vi "SwerveMath_.vi"(2 "Rotation Multipliers":dbl, 3 "Trigger Axes/Turn Speed":cluster{"Left":dbl, "Right":dbl}, 4 "Strafe Multiplier":dbl, 5 "Angle (radians; 0 = right)":dbl, 6 "FieldCentric? (T)":bool=TRUE, 7 "Strafe Joystick Axes":cluster{"X":dbl, "Y":dbl}) -> (0 "Motor Angles":dbl[](array[numeric]), 1 "Motor Speeds":dbl[](array[numeric]))   [LabVIEW 2015]
uses:
  Swerve Drive Published Globals.vi
panel:
  in  "Rotation Angle Cluster":dbl
  in  "Rotation Multiplier":dbl
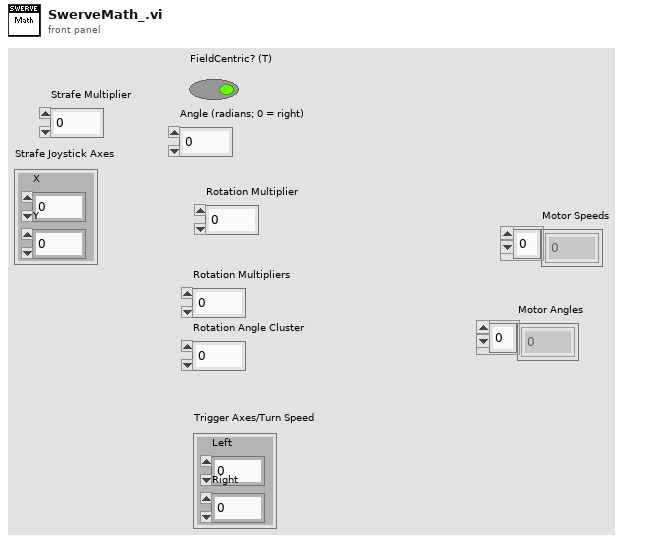
[diagram p1: front panel]
types:
  T1 = cluster{"FL Angle":dbl, "FR Angle":dbl, "RL Angle":dbl, "RR Angle":dbl}
  T2 = cluster{"normalized array[0]":dbl, "normalized array[1]":dbl, "normalized array[2]":dbl, "normalized array[3]":dbl}
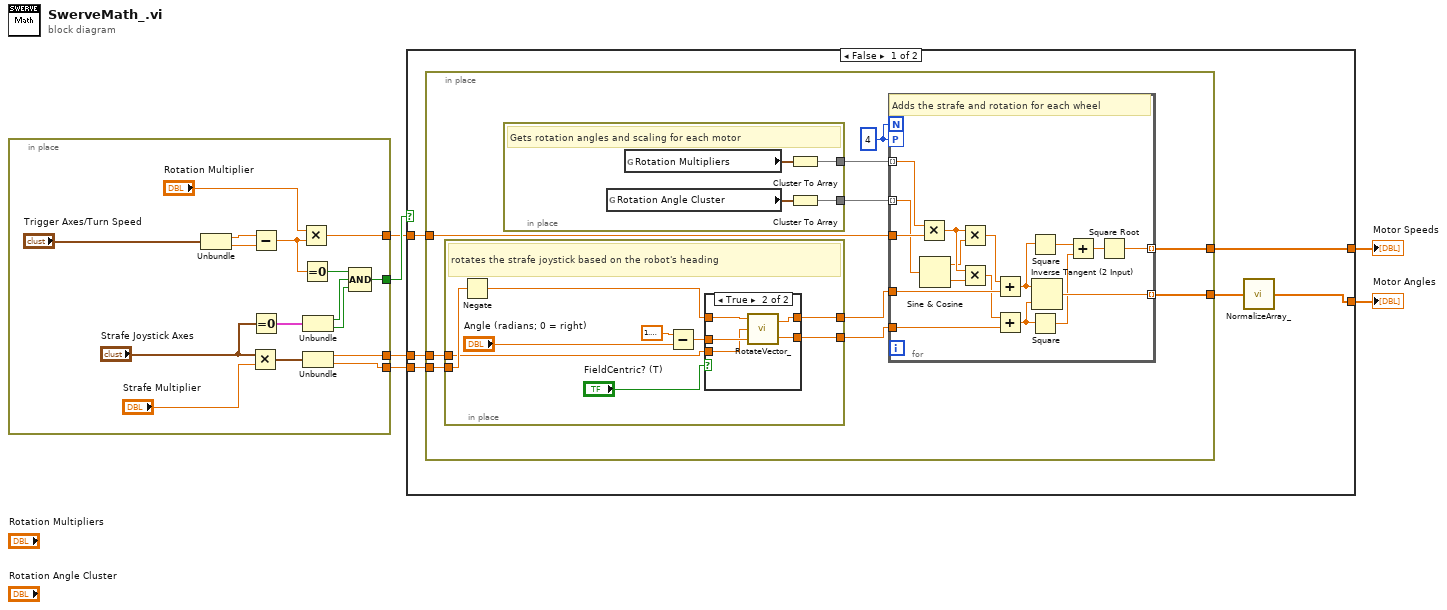
[diagram p0: block diagram]
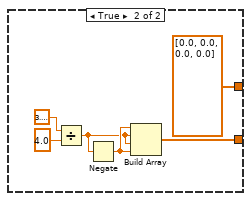
[diagram p3: hidden frame]
diagram:
  n1 = in-place {
    in-place-border: [w15] -> w6
    in-place-border: [w14] -> w5
    in-place-border: [w13] -> w4
    in-place-border: [w11] -> w3
    n2 = Unbundle("Trigger Axes/Turn Speed") -> ("Left"=w18:dbl, "Right"=w19:dbl)
    n3 = Multiply(x="Strafe Joystick Axes", y="Strafe Multiplier") -> (x*y=w9:cluster{"X":dbl, "Y":dbl})
    n4 = Subtract(x=w18, y=w19) -> (x-y=w12:dbl)
    n5 = Equal To 0?(x="Strafe Joystick Axes") -> (x = 0?=w21:cluster{"X":bool, "Y":bool})
    n6 = Multiply(x="Rotation Multiplier", y=w12) -> (x*y=w11:dbl)
    n7 = Equal To 0?(x=w12) -> (x = 0?=w7:bool)
    n8 = Unbundle(w21) -> ("X"=w17:bool, "Y"=w16:bool)
    n9 = Unbundle(w9) -> ("X"=w13:dbl, "Y"=w14:dbl)
    n10 = Compound Arithmetic op=AND(w7, w17, w16) -> (w15:bool)
  }
  n11 = case shown="False" w6 {
    tunnel: w5 -> [w28 _]
    tunnel: w4 -> [w27 _]
    tunnel: w3 -> [w26 _]
    tunnel: [w25 dbl[] [0.0, 0.0, 0.0, 0.0] ("appended array")] -> w2
    tunnel: [w23 w76] -> w1
    frame False {
      n12 = in-place {
        in-place-border: [w36] -> w25
        in-place-border: [w35] -> w24
        in-place-border: w28 -> [w33]
        in-place-border: w27 -> [w32]
        in-place-border: w26 -> [w31]
        w34 = 4
        n13 = in-place {
          in-place-border: [w51] -> w38
          in-place-border: [w50] -> w37
          in-place-border: w33 -> [w46]
          in-place-border: w32 -> [w45]
          # "rotates the strafe joystick based on the robot's heading"
          n14 = Negate(x=w46) -> (-x=w47:dbl)
          n15 = Subtract(x=1.5707963267948966, y="Angle (radians; 0 = right)") -> (x-y=w48:dbl)
          n16 = case shown="True" "FieldCentric? (T)" {
            tunnel: w47 -> [w53 w58]
            tunnel: [w53 w55] -> w51
            tunnel: [w52 w54] -> w50
            tunnel: w48 -> [_ w57]
            tunnel: w45 -> [w52 w56]
            frame False {
            }
            frame True {
              n17 = call "RotateVector_.vi"("Angle"=w57, "X"=w56, "Y"=w58) -> ("X'"=w54:dbl, "Y'"=w55:dbl)
            }
          }
        }
        n18 = in-place {
          in-place-border: [w41] -> w30
          in-place-border: [w42] -> w29
          # "Gets rotation angles and scaling for each motor"
          n19 = global read "Swerve Drive Published Globals.vi" "Rotation Angle Cluster"() -> (w39:T1)
          n20 = global read "Swerve Drive Published Globals.vi" "Rotation Multipliers"() -> (w40:T2)
          n21 = Cluster To Array(cluster=w40) -> (array=w41:dbl[])
          n22 = Cluster To Array(cluster=w39) -> (array=w42:dbl[])
        }
        n23 = for {
          N: w34 -> [_]
          tunnel: w38 -> [w75]
          tunnel: w37 -> [w74]
          tunnel: w31 -> [w73]
          tunnel: [w72] -> w36 mode=indexing
          tunnel: [w71] -> w35 mode=indexing
          workers-P: w34 -> [_]
          tunnel: w30 -> [w60] mode=indexing
          tunnel: w29 -> [w59] mode=indexing
          # "Adds the strafe and rotation for each wheel"
          n24 = Multiply(x=w60, y=w73) -> (x*y=w63:dbl)
          n25 = Sine & Cosine(0:w59) -> (1:w62:dbl, 2:w61:dbl)
          n26 = Multiply(x=w63, y=w62) -> (x*y=w66:dbl)
          n27 = Multiply(x=w63, y=w61) -> (x*y=w67:dbl)
          n28 = Add(x=w66, y=w75) -> (x+y=w65:dbl)
          n29 = Add(x=w67, y=w74) -> (x+y=w64:dbl)
          n30 = Square(x=w65) -> (x^2=w69:dbl)
          n31 = Square(x=w64) -> (x^2=w68:dbl)
          n32 = Inverse Tangent (2 Input)(1:w64, 2:w65) -> (0:w71:dbl)
          n33 = Add(x=w69, y=w68) -> (x+y=w70:dbl)
          n34 = Square Root(x=w70) -> (sqrt(x)=w72:dbl)
        }
      }
      n35 = call "NormalizeArray_.vi"("array"=w24) -> ("normalized array"=w23:dbl[])
    }
    frame True {
      n36 = Divide(x=3.141592653589793, y=4.0) -> (x/y=w80:dbl)
      n37 = Negate(x=w80) -> (-x=w81:dbl)
      n38 = Build Array(w81, w80, w80, w81) -> (w76:dbl[])
    }
  }
  "Motor Speeds" <- w2
  "Motor Angles" <- w1
